vi "RunTest2.vi"(8 "error in (no error)":errorcluster, 11 "Prueba09 in":refnum<class "Prueba09.lvclass">) -> (0 "error out":errorcluster, 2 "resultado":string, 3 "Prueba09 out":refnum<class "Prueba09.lvclass">)   [LabVIEW 2019]
uses:
  <vilib>/Utility/miscctls.llb/LVRowAndColumnTypeDef.ctl
  Prueba/Prueba.lvclass
  Controles/Estados_P09.ctl
  Prueba09.lvclass
  Controles/MessageP09.ctl
  QMH/User Event - Stop/User Event - Stop.lvlib
  QMH/Message Queue/Message Queue.lvlib
  QMH/Message Queue/Enqueue Message (Single).vi
  ClusterGEN.ctl
  Prueba04/Control/Slide.ctl
  Prueba04/Prueba04.lvclass
  <vilib>/Utility/error.llb/Error Cluster From Error Code.vi
  <vilib>/ErrorRing/Error Ring.xnode
  <vilib>/Utility/error.llb/DialogType.ctl
  D:/REPO/GitHub/procal/Pruebas/Prueba/Prueba.lvclass
panel:
  out "elapsed time":dbl
  out "cuenta":i32
  out "tablaPeakRef[dB]":string[](array[string])
  out "Vref2":dbl
  out "Pict Ring 2":u16(ring)
  out "Pict Ring 3":u16(ring)
  out "cumple_no_cumple":bool
  out "Vref":dbl
  in  "Tab":enum32{"Page 1", "Page 2", "Page 3"}(tab)
  out "NivMaxCpeak":dbl=140.0
  out "NivelRMSensayo":dbl=95.0
  out "frecuencia1":dbl=140.0
  in  "guardar_Vref":bool
  in  "generar1":bool
  in  "AjusteAmp":T1 caption="Ajuste de amplitud [mV]" scale=0.0..100.0
  out "voltMon1":dbl format="%#.1f"
  out "frecMon1":dbl format="%#.1f"
  in  "seguir":bool
  out "NivMaxCpeak2":dbl=140.0
  out "NivelRMSensayo2":dbl=95.0
  out "frecuencia2":dbl=140.0
  in  "guardar_Vref2":bool
  in  "generar2":bool
  in  "AjusteAmp2":T1 caption="Ajuste de amplitud [mV]" scale=0.0..100.0
  out "voltMon2":dbl format="%#.1f"
  out "frecMon2":dbl format="%#.1f"
  in  "seguir2":bool
  out "Pict Ring 4":u16(ring)
  out "Pict Ring 1":u16(ring)
  out "led":bool
  in  "knobFrec":dbl(knob)=1.0 min=1.0 max=3.0 scale=1.0..3.0
  in  "genera3":bool caption="PruebaSup"
  out "voltMon500":dbl format="%#.1f"
  out "nivelRMS500":dbl format="%#.1f"
  in  "Tabla":string[][](table)
  in  "salir":bool
  out "cumple":bool
  out "no_cumple":bool
  out "voltMon8000":dbl format="%#.1f"
  out "nivelRM8000":dbl format="%#.1f"
  # "Selección de Señal de referencia 8000 Hz"
  # "Elección Señal de Referencia\nsegún marca y modelo de sonómetro"
  # "Nivel RMS para Ensayo"
  # "Nivel Máximo Cpeak"
  # "Frecuencia"
  # "Monitoreo"
  # "Frecuencia"
  # "Hz"
  # "Voltaje"
  # "mV"
  # "9. Nivel de sonido con ponderación Cpeak. IEC 61672-3: 2006 Cláusula 17"
  # "Selección de Señal de referencia 500 Hz"
  # "Elección Señal de Referencia\nsegún marca y modelo de sonómetro"
  # "Nivel RMS para Ensayo"
  # "Nivel Máximo Cpeak"
  # "Frecuencia"
  # "Monitoreo"
  # "Frecuencia"
  # "Hz"
  # "Voltaje"
  # "mV"
  # "9. Nivel de sonido con ponderación Cpeak. IEC 61672-3: 2006 Cláusula 17"
  # "Tabla Resultados"
  # "Genera peak"
  # "Cumple"
  # "No Cumple"
  # "500 Hz"
  # "Nivel RMS para Ensayo"
  # "dB"
  # "Voltaje"
  # "mV"
  # "9. Nivel de sonido con ponderación Cpeak. IEC 61672-3: 2006 Cláusula 17"
  # "8000 Hz"
  # "Nivel RMS para Ensayo"
  # "dB"
  # "Voltaje"
  # "mV"
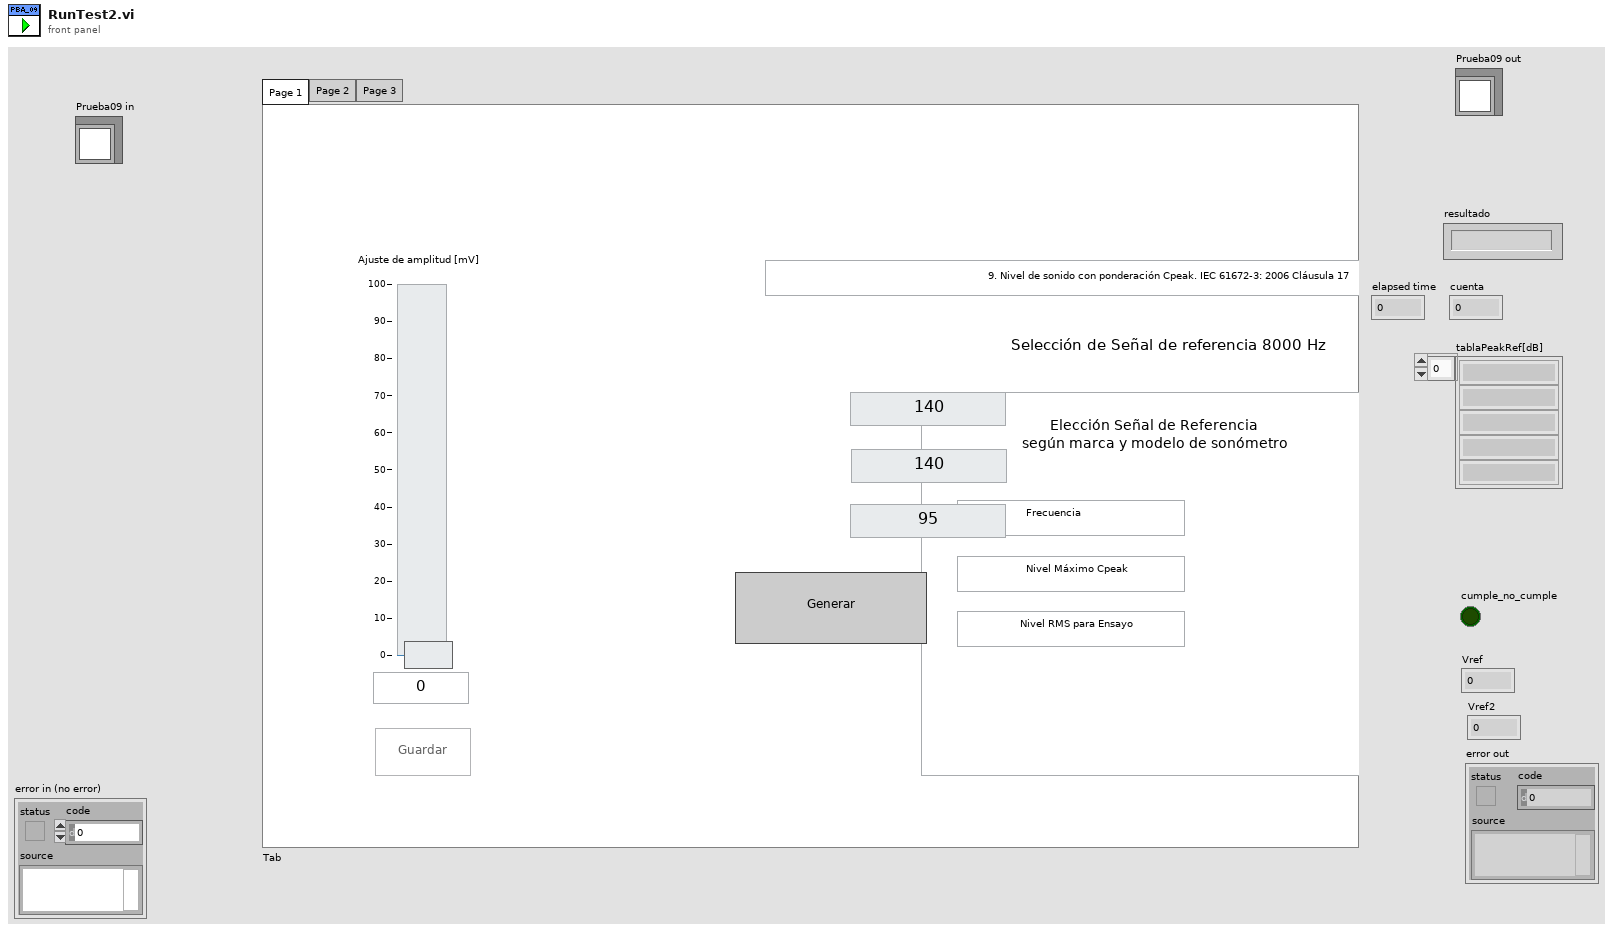
[diagram p1: front panel]
types:
  T1 = typedef "Prueba04.lvclass/Slide.ctl" = dbl
  T2 = typedef "LVRowAndColumnTypeDef.ctl" = cluster{"Row":i32, "Column":i32}
  T3 = typedef "Message Queue.lvlib/All Message Queues.ctl" = cluster{"MHL":refnum<queue>, "Inst_CNT90":refnum<queue>, "Inst_DS360":refnum<queue>, "Inst_Keithley2002":refnum<queue>, "Inst_DAQ":refnum<queue>, "BD":refnum<queue>, "Pistofono":refnum<queue>, "Nexus":refnum<queue>}
  T4 = enum8{"Enabled", "Disabled", "Disabled and Grayed Out"}
  T5 = enum32{"Page 1", "Page 2", "Page 3", "Page 4", "Page 5", "Page 6", "Page 7"}
  T6 = typedef "Prueba09.lvclass/ClusterGEN.ctl" = cluster{"frec":dbl, "amp":dbl, "tipo_ciclo":string}
  T7 = cluster{"ControlName":string, "ControlReference":refnum<vi>}[]
  T8 = typedef "Prueba09.lvclass/MessageP09.ctl" = cluster{"Estados":T9, "Data":variant}
  T9 = typedef "Prueba09.lvclass/Estados_P09.ctl" = enum16{"Error", "DetieneInstrumentos", "InicializarInstrumentos", "LeerArchivoConfiguracion", "inicio", "configurarTabla", "FrecAmp1", "FrecAmp2", "FrecAmp3", "iniciarGEN", "iniciaGEN_Peak", "detenerGEN", "guardaVref", "guardaVref2", "monitoreo", "peakRefer", "ingresaMediciones", "guardaMediciones", "cumplimiento", "listo_evaluar", "evaluar", "final", "salir"}
  T10 = typedef "DialogType.ctl" = u16
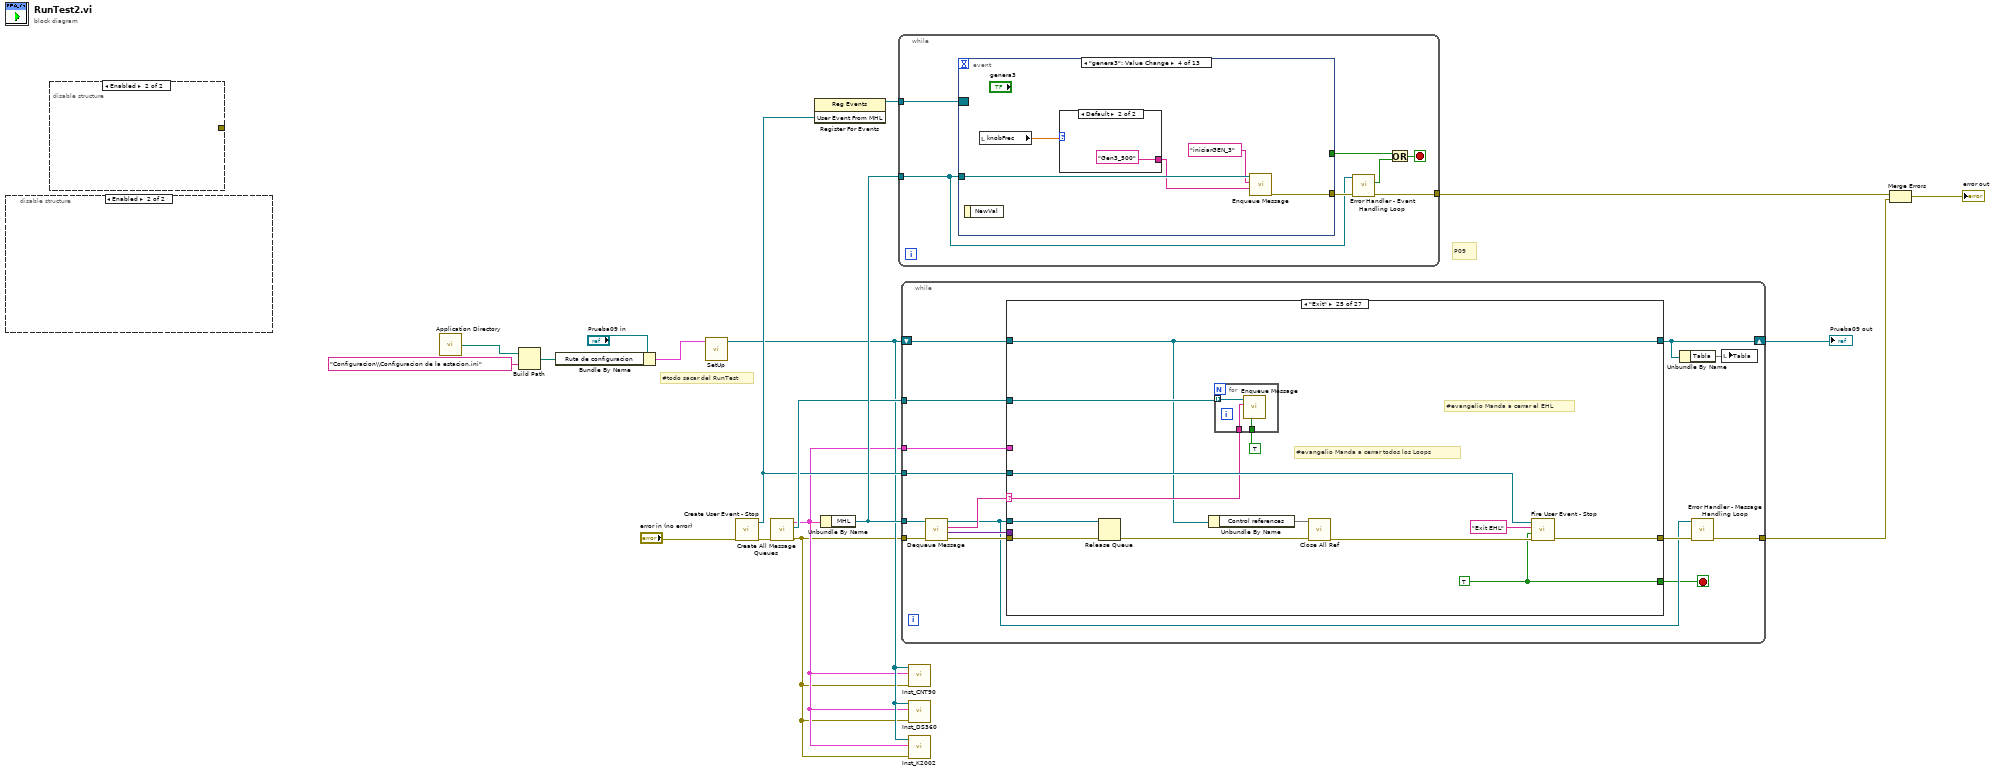
[diagram p0: block diagram]
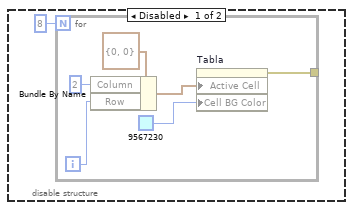
[diagram p2: hidden frame]
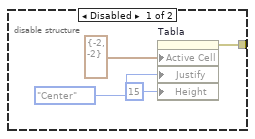
[diagram p3: hidden frame]
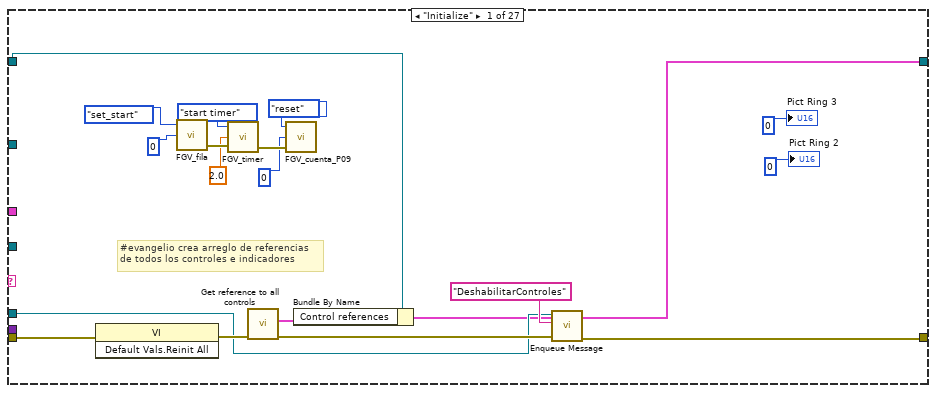
[diagram p4: hidden frame]
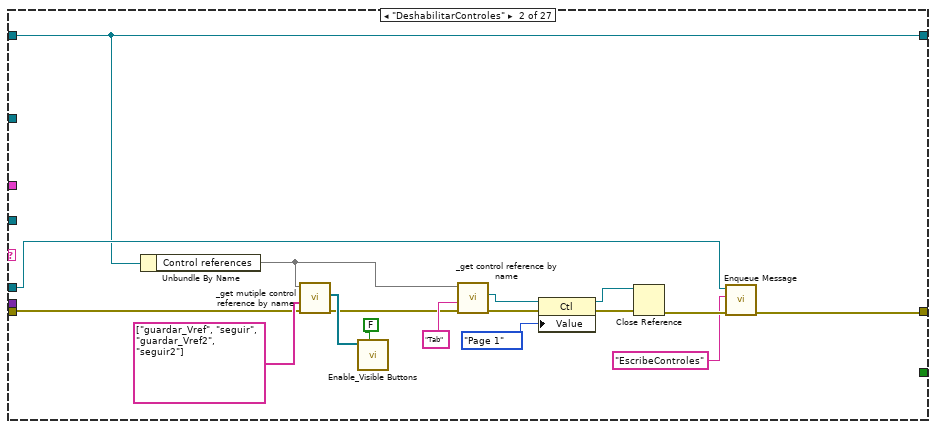
[diagram p5: hidden frame]
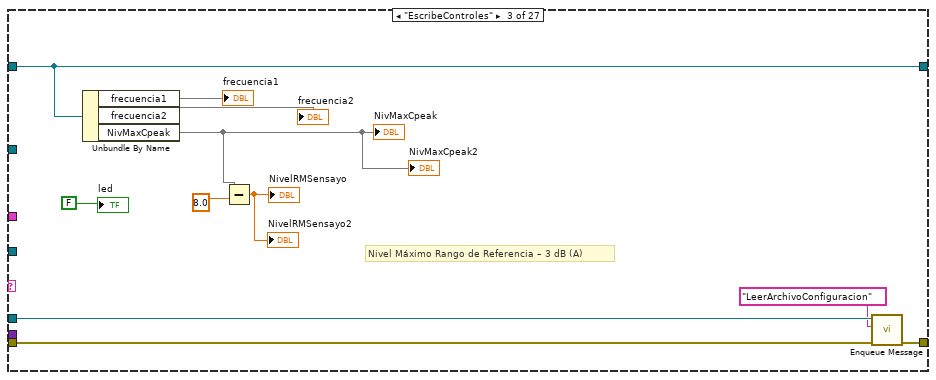
[diagram p6: hidden frame]
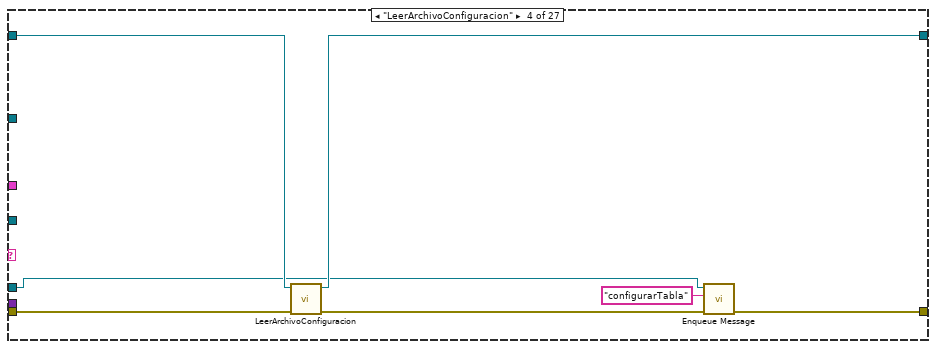
[diagram p7: hidden frame]
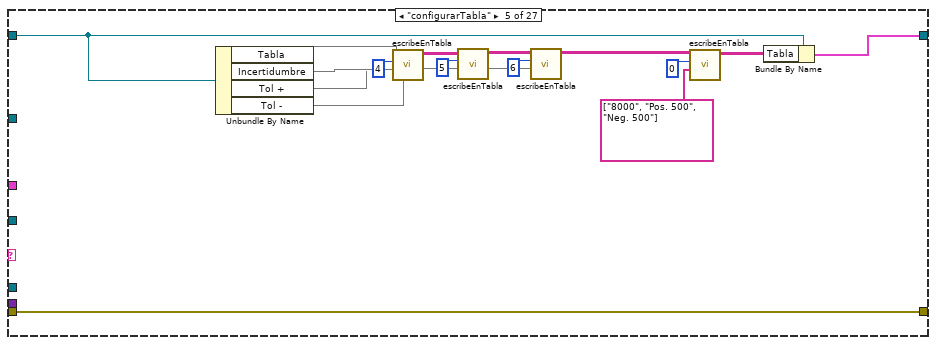
[diagram p8: hidden frame]
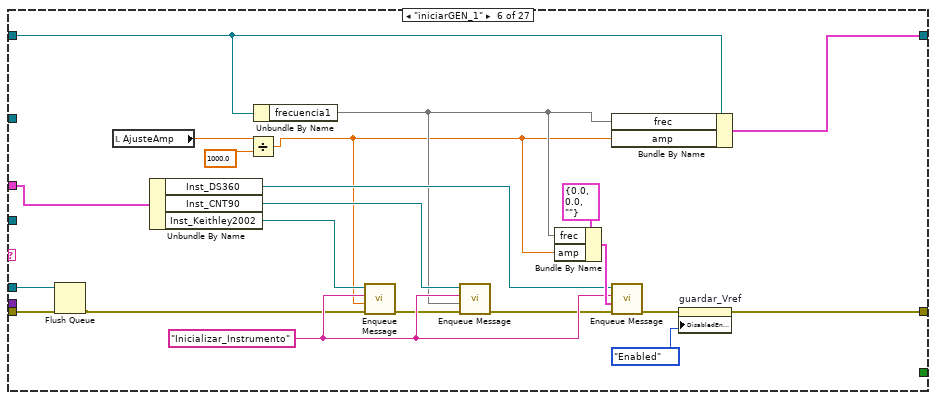
[diagram p9: hidden frame]
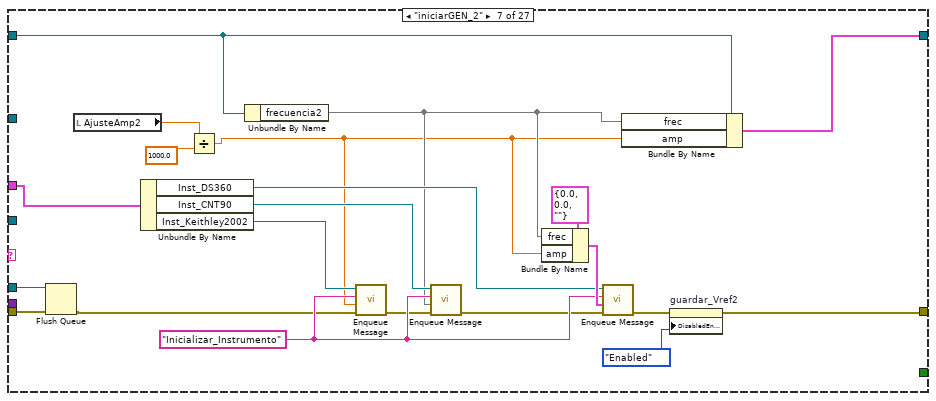
[diagram p10: hidden frame]
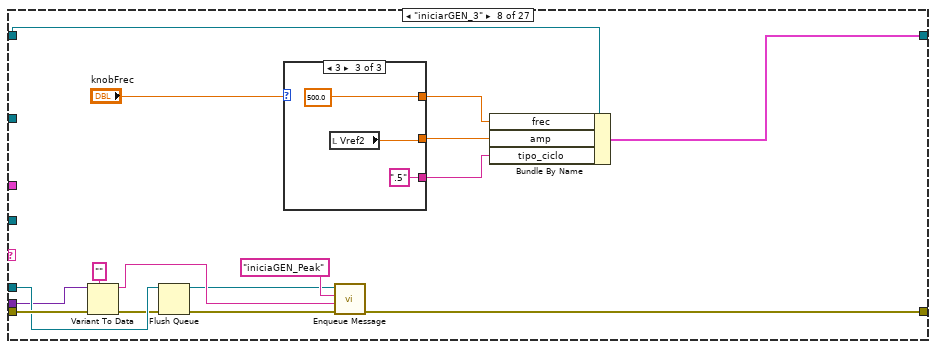
[diagram p11: hidden frame]
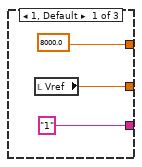
[diagram p12: hidden frame]
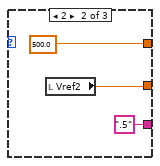
[diagram p13: hidden frame]
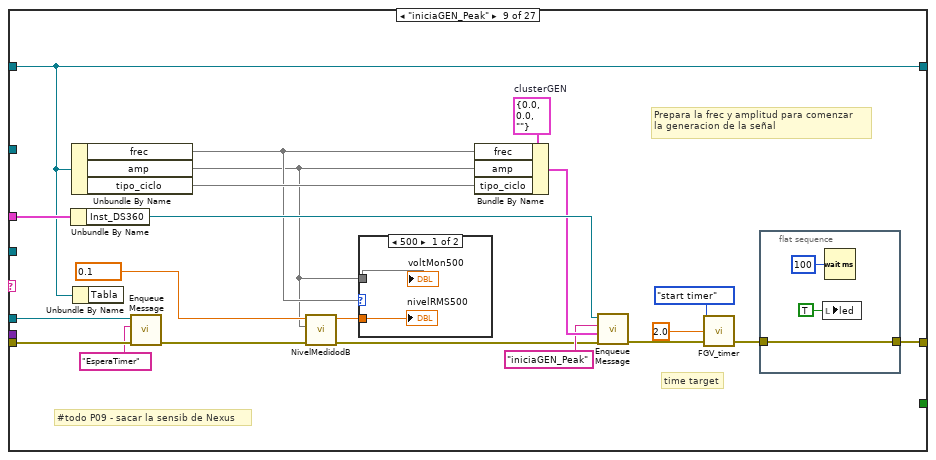
[diagram p14: hidden frame]
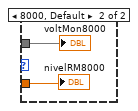
[diagram p15: hidden frame]
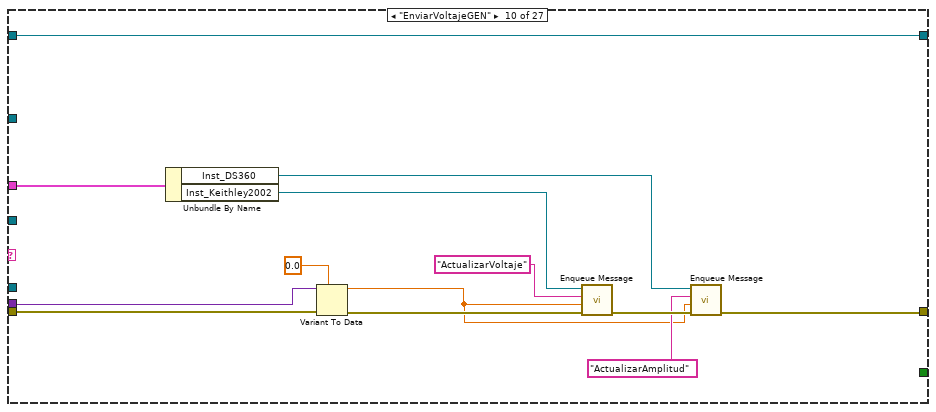
[diagram p16: hidden frame]
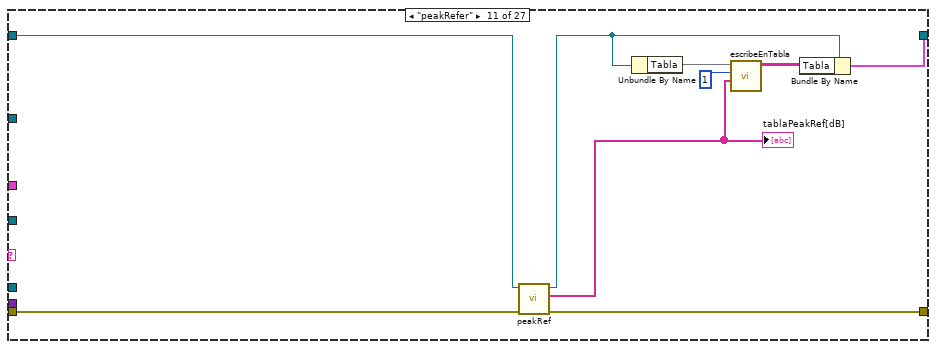
[diagram p17: hidden frame]
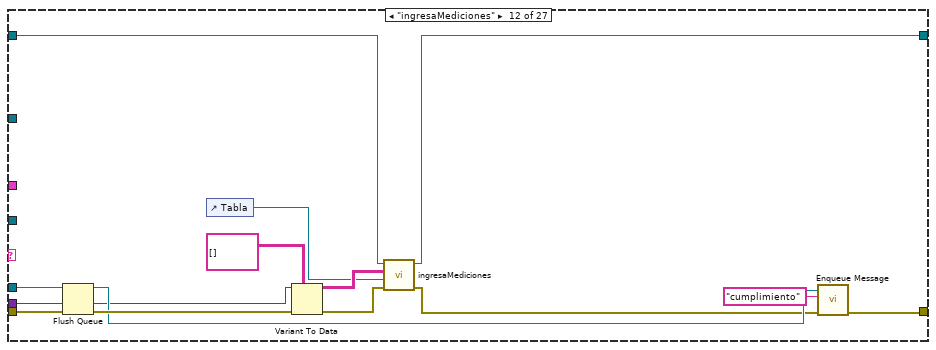
[diagram p18: hidden frame]
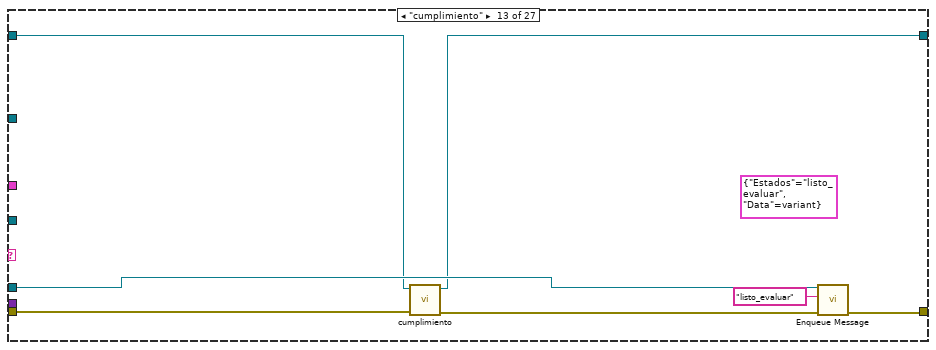
[diagram p19: hidden frame]
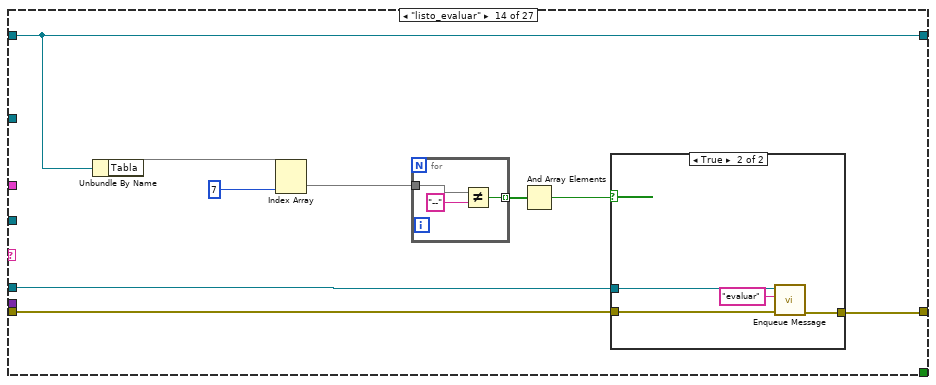
[diagram p20: hidden frame]
diagram:
  # "P09"
  # "#todo sacar del RunTest"
  n1 = disable-structure shown="Enabled" {
    frame Disabled {
      n2 = for {
        N: 8 -> [_]
        tunnel: [w21] -> _
        i -> [w20]
        n3 = Bundle By Name(cluster=T2 {"Row"=0, "Column"=0} ("Active Cell:Active Cell"), "Column"=2, "Row"=w20) -> (w23:T2)
        n4 = property on="Tabla" class="Tbl (strict)"("Active Cell"=w23, "Cell BG Color"=u32 9567230) -> (error out=w21:errorcluster)  [unwired: 2 in, 1 out]
      }
    }
    frame Enabled {
    }
  }
  n5 = disable-structure shown="Enabled" {
    disable-tunnel: [w28 _] -> _
    frame Disabled {
      n6 = property on="Tabla" class="Tbl (strict)"("Active Cell"=T2 {"Row"=-2, "Column"=-2} ("Active Cell:Active Cell"), "Justify"=enum16{"Left", "Center", "Right"}."Center" ("Active Cell:Cell Justification"), "Height"=u32 15 ("Active Cell:Cell Font:Size")) -> (error out=w28:errorcluster)  [unwired: 2 in, 1 out]
    }
    frame Enabled {
    }
  }
  n7 = call <vilib>:"Application Directory.vi"() -> ("Application Directory"=w14:path)
  n8 = Build Path(base path=w14, name or relative path="Configuracion\\Configuracion de la estacion.ini") -> (appended path=w11:path)
  n9 = Bundle By Name(cluster="Prueba09 in", "Ruta de configuracion"=w11) -> (w12:cluster{})
  n10 = call-dynamic "SetUp.vi"("Prueba08 in"=w12) -> ("Prueba08 out"=w3:refnum<class "Prueba09.lvclass">)  [unwired: 9 in, 1 out]
  n11 = call "Create User Event - Stop.vi"("error in (no error)"="error in (no error)") -> ("error out"=w9:errorcluster, "User Event From MHL"=w4:refnum<user-event>)  [unwired: 9 in]
  n12 = call "Create All Message Queues.vi"("error in (no error)"=w9) -> ("error out"=w1:errorcluster, "PL Queues Array"=w5:refnum<queue>[], "All Message Queues out"=w2:T3)  [unwired: 8 in]
  n13 = register-events(w4) -> (reference out=w6:refnum<event-registration>)  [unwired: 2 in, 1 out]
  n14 = Unbundle By Name(w2) -> ("MHL"=w7:refnum<queue>)
  n15 = while {
    tunnel: w7 -> [w31]
    tunnel: [w33] -> w18
    tunnel: w6 -> [w35]
    stop <- w36 stop-if-true
    n16 = event shown="[3] \"genera3\": Value Change" {
      selector: w35 -> [_ _ _ _ _ _ _ _ _ _ _ _ _]
      dyn-events: _ -> [_ _ _ _ _ _ _ _ _ _ _ _ _]
      timeout: _ -> [_ _ _ _ _ _ _ _ _ _ _ _ _]
      tunnel: w31 -> [w39 w44 w51 w55 _ w65 w70 w72 w81 w87 w91 _ w99]
      tunnel: [w38 w45 w50 w56 w60 w61 w71 w74 w78 w83 w90 _ _] -> w34
      tunnel: [_ _ _ _ _ _ _ _ _ _ _ w92 _] -> w30
      event "salir": Value Change {
        n17 = event-data() -> ()  [unwired: 1 in, 1 out]
        n18 = call-poly "Enqueue Message.vi"("Message"="Exit", "Message Queue"=w39) -> ("error out"=w38:errorcluster)  [unwired: 8 in, 1 out]
      }
      event "generar1": Value Change {
        n19 = event-data() -> ("NewVal"=w41:bool)  [unwired: 1 in]
        n20 = Select(t="iniciarGEN_1", s=w41, f="detenerGEN") -> (s? t:f=w40:string)
        n21 = call-poly "Enqueue Message.vi"("Message"=w40, "Message Queue"=w44) -> ("error out"=w45:errorcluster)  [unwired: 8 in, 1 out]
      }
      event "generar2": Value Change {
        n22 = event-data() -> ("NewVal"=w48:bool)  [unwired: 1 in]
        n23 = Select(t="iniciarGEN_2", s=w48, f="detenerGEN") -> (s? t:f=w46:string)
        n24 = call-poly "Enqueue Message.vi"("Message"=w46, "Message Queue"=w51) -> ("error out"=w50:errorcluster)  [unwired: 8 in, 1 out]
      }
      event "genera3": Value Change {
        n25 = event-data() -> ()  [unwired: 1 in, 1 out]
        n26 = local read "knobFrec"() -> (w54:dbl)
        n27 = case shown="Default" w54 {
          tunnel: ["Gen3_8000" "Gen3_500"] -> w52
          frame 1 {
          }
          frame Default {
          }
        }
        n28 = call-poly "Enqueue Message.vi"("Message Data"=w52, "Message"="iniciarGEN_3", "Message Queue"=w55) -> ("error out"=w56:errorcluster)  [unwired: 7 in, 1 out]
      }
      event "seguir": Value Change {
        n29 = event-data() -> ()  [unwired: 1 in, 1 out]
        n30 = property on="Tab" class="TabCtl (strict)"("Value"=enum32{"Page 1", "Page 2", "Page 3"}."Page 2" ("Tab")) -> (error out=w60:errorcluster)  [unwired: 2 in, 1 out]
      }
      event "seguir2": Value Change {
        n31 = event-data() -> ()  [unwired: 1 in, 1 out]
        n32 = call-poly "Enqueue Message.vi"("Message"="peakRefer", "Message Queue"=w65) -> ("error out"=w62:errorcluster)  [unwired: 8 in, 1 out]
        n33 = property on="Tab" class="TabCtl (strict)"(error in=w62, "Value"=enum32{"Page 1", "Page 2", "Page 3"}."Page 3" ("Tab")) -> (error out=w61:errorcluster)  [unwired: 1 in, 1 out]
      }
      event Value Change {
        n34 = event-data() -> ()  [unwired: 1 in, 1 out]
        n35 = Divide(x="AjusteAmp", y=T1 1000.0) -> (x/y=w66:T1)
        n36 = call-poly "Enqueue Message.vi"("Message Data"=w66, "Message"="EnviarVoltajeGEN", "Message Queue"=w70) -> ("error out"=w71:errorcluster)  [unwired: 7 in, 1 out]
      }
      event Value Change {
        n37 = event-data() -> ()  [unwired: 1 in, 1 out]
        n38 = Divide(x="AjusteAmp2", y=T1 1000.0) -> (x/y=w75:T1)
        n39 = call-poly "Enqueue Message.vi"("Message Data"=w75, "Message"="EnviarVoltajeGEN", "Message Queue"=w72) -> ("error out"=w74:errorcluster)  [unwired: 7 in, 1 out]
      }
      event "guardar_Vref": Value Change {
        n40 = event-data() -> ()  [unwired: 1 in, 1 out]
        n41 = call-poly "Enqueue Message.vi"("Message"="guardaVref", "Message Queue"=w81) -> ("error out"=w79:errorcluster)  [unwired: 8 in, 1 out]
        n42 = property on="seguir" class="Bool"(error in=w79, "DisabledEnum"=T4."Enabled" ("Disabled")) -> (error out=w78:errorcluster)  [unwired: 1 in, 1 out]
      }
      event "guardar_Vref2": Value Change {
        n43 = event-data() -> ()  [unwired: 1 in, 1 out]
        n44 = call-poly "Enqueue Message.vi"("Message"="guardaVref2", "Message Queue"=w87) -> ("error out"=w84:errorcluster)  [unwired: 8 in, 1 out]
        n45 = property on="seguir2" class="Bool"(error in=w84, "DisabledEnum"=T4."Enabled" ("Disabled")) -> (error out=w83:errorcluster)  [unwired: 1 in, 1 out]
      }
      event "Tabla": Value Change {
        n46 = event-data() -> ("NewVal"=w89:string[][])  [unwired: 1 in]
        n47 = call-poly "Enqueue Message.vi"("Message Data"=w89, "Message"="ingresaMediciones", "Message Queue"=w91) -> ("error out"=w90:errorcluster)  [unwired: 7 in, 1 out]
      }
      event User Event {
        n48 = event-data() -> ("User Event"=w94:string, "Event Data"=w93:variant)  [unwired: 1 in]
        n49 = case shown="\"Exit EHL\"" w94 {
          tunnel: w93 -> [_ w96]
          tunnel: [_ w95] -> w92
          frame Default {
          }
          frame "Exit EHL" {
            # "#evangelio Termina\nla ejecucion del EHL"
            n50 = Variant To Data(type=TRUE, Variant=w96) -> (data=w95:bool)  [unwired: 1 in, 1 out]
          }
        }
      }
      event Panel Close? {
        w98 = TRUE
        n51 = event-data() -> ()  [unwired: 1 in, 1 out]
        n52 = call-poly "Enqueue Message.vi"("Priority Message? (F)"=w98, "Message"="Confirmar Salida", "Message Queue"=w99) -> ()  [unwired: 7 in, 2 out]
        n53 = event-data("Discard?"=w98) -> ()  [unwired: 1 in, 1 out]
      }
    }
    n54 = call "Error Handler - Event Handling Loop.vi"("error in (no error)"=w34, "Message Queue"=w31) -> ("dup error in"=w33:errorcluster, "Error?"=w32:bool)  [unwired: 7 in, 1 out]
    n55 = Or(x=w30, y=w32) -> (x .or. y?=w36:bool)
  }
  n56 = while {
    tunnel: w7 -> [w109]
    tunnel: w1 -> [w108]
    tunnel: [w103] -> w10
    shift-right: [w114] -> w16
    shift-left: w3 -> [w115]
    tunnel: w2 -> [w112]
    tunnel: w5 -> [w111]
    tunnel: w4 -> [w110]
    stop <- w101 stop-if-true
    n57 = call "Dequeue Message.vi"("error in (no error)"=w108, "Message Queue"=w109) -> ("error out"=w107:errorcluster, "Message Data"=w105:variant, "Message"=w106:string, "dup Message Queue"=w102:refnum<queue>)  [unwired: 6 in]
    n58 = case shown="\"Exit\"" w106 {
      selector: w106 -> [_ _ _ _ _ _ _ _ _ _ _ _ _ _ _ _ _ _ _ _ _ _ _ _ w470 _ w497]
      tunnel: w105 -> [_ _ _ _ _ _ _ w233 _ w283 _ w310 _ _ _ _ _ w407 w416 _ _ _ w455 _ _ _ _]
      tunnel: w107 -> [w129 w138 w162 w169 w179 w195 w215 w243 w273 w284 w302 w316 w323 w332 w348 w359 w363 w408 w417 w422 w441 w448 w458 w466 w474 w485 _]
      tunnel: [w128 w135 w161 w165 w179 w193 w211 w242 w268 w281 w301 w315 w321 w331 w346 w359 w374 w402 w412 w418 w441 w448 w456 w466 w468 w483 w496] -> w104
      tunnel: w102 -> [w130 w137 w160 w164 _ w194 w214 w240 w260 _ _ w313 w320 w330 w347 _ w362 _ _ w421 _ _ w457 _ w473 w484 _]
      tunnel: w115 -> [w117 w136 w158 w167 w176 w205 w226 w238 w255 w293 w300 w308 w319 w325 w343 w354 w361 w406 w415 w419 w442 w449 w464 w465 w469 w490 w498]
      tunnel: [w116 w136 w158 w168 w175 w206 w227 w239 w255 w293 w295 w307 w318 w325 w343 w354 w361 w405 w414 w419 w442 w449 w464 w465 w469 w490 w498] -> w114
      tunnel: w112 -> [_ _ _ _ _ w192 w213 _ w267 w282 _ _ _ _ _ _ _ _ _ w420 _ _ _ _ _ _ _]
      tunnel: w111 -> [_ _ _ _ _ _ _ _ _ _ _ _ _ _ _ _ _ _ _ _ _ _ _ _ w472 _ _]
      tunnel: w110 -> [_ _ _ _ _ _ _ _ _ _ _ _ _ _ _ _ _ _ _ _ _ _ _ _ w471 _ _]
      tunnel: [_ _ _ _ _ _ _ _ _ _ _ _ _ _ _ _ _ _ _ _ _ _ _ _ w467 _ _] -> w101
      frame "Initialize" {
        # "#evangelio crea arreglo de referencias\nde todos los controles e indicadores"
        n59 = invoke class="VI" method="Default Vals.Reinit All"(error in=w129) -> (error out=w133:errorcluster)  [unwired: 2 in, 2 out]
        n60 = call "FGV_fila.vi"("fila_inicial"=0, "action"=enum16{"increment", "set_start", "get"}."set_start") -> ("error out"=w127:errorcluster)  [unwired: 2 in, 1 out]
        n61 = call "FGV_timer.vi"("error in (no error)"=w127, "time target"=2.0, "action"=enum16{"get time", "start timer"}."start timer") -> ("error out"=w126:errorcluster)  [unwired: 2 out]
        n62 = call "Get reference to all controls.vi"("error in (no error)"=w133) -> ("error out"=w131:errorcluster, "Control references"=w132:T7)  [unwired: 5 in]
        n63 = call "FGV_cuenta_P09.vi"("error in (no error)"=w126, "cuenta in"=0, "action"=enum16{"increment", "reset", "get"}."reset") -> ()  [unwired: 1 in, 2 out]
        n64 = Bundle By Name(cluster=w117, "Control references"=w132) -> (w116:cluster{})
        n65 = call-poly "Enqueue Message.vi"("error in (no error)"=w131, "Message"="DeshabilitarControles", "Message Queue"=w130) -> ("error out"=w128:errorcluster)  [unwired: 7 in, 1 out]
        "Pict Ring 2" <- u16 0 ("Pict Ring 2")
        "Pict Ring 3" <- u16 0 ("Pict Ring 3")
      }
      frame "DeshabilitarControles" {
        n66 = Unbundle By Name(w136) -> ("Control references"=w147)
        n67 = call "_get mutiple control reference by name.vi"("error in (no error)"=w138, "Control names"=string[] ["guardar_Vref", "seguir", "guardar_Vref2", "seguir2"], "Control references"=w147) -> ("error out"=w144:errorcluster, "References"=w145:refnum<vi>[])  [unwired: 3 in]
        n68 = call "Enable_Visible Buttons.vi"("Enable? (T)"=FALSE, "Controls Ref Array"=w145) -> ()  [unwired: 10 in]
        n69 = call "_get control reference by name.vi"("error in (no error)"=w144, "Control name"="Tab" ("Message"), "Control references"=w147) -> ("error out"=w151:errorcluster, "Ctl Refnum"=w149:refnum<vi>)  [unwired: 3 in]
        n70 = property class="Ctl"(reference=w149, error in=w151, "Value"=T5."Page 1" ("Tab_Prueba04")) -> (reference out=w140:refnum<vi>, error out=w142:errorcluster)
        n71 = Close Reference(reference=w140, error in (no error)=w142) -> (error out=w141:errorcluster)
        n72 = call-poly "Enqueue Message.vi"("error in (no error)"=w141, "Message"="EscribeControles", "Message Queue"=w137) -> ("error out"=w135:errorcluster)  [unwired: 7 in, 1 out]
      }
      frame "EscribeControles" {
        # "Nivel Máximo Rango de Referencia – 3 dB (A)"
        n73 = Unbundle By Name(w158) -> ("frecuencia1"=→"frecuencia1", "frecuencia2"=→"frecuencia2", "NivMaxCpeak"=w155)
        "NivMaxCpeak" <- w155
        "NivMaxCpeak2" <- w155
        n74 = Subtract(x=w155, y=8.0) -> (x-y=→"NivelRMSensayo" →"NivelRMSensayo2":dbl)
        n75 = call-poly "Enqueue Message.vi"("error in (no error)"=w162, "Message"="LeerArchivoConfiguracion", "Message Queue"=w160) -> ("error out"=w161:errorcluster)  [unwired: 7 in, 1 out]
        "led" <- FALSE ("led")
      }
      frame "LeerArchivoConfiguracion" {
        n76 = call "LeerArchivoConfiguracion.vi"("error in"=w169, "Prueba31 in"=w167) -> ("error out"=w166:errorcluster, "Prueba31 out"=w168:refnum<class "Prueba09.lvclass">)  [unwired: 8 in]
        n77 = call-poly "Enqueue Message.vi"("error in (no error)"=w166, "Message"="configurarTabla", "Message Queue"=w164) -> ("error out"=w165:errorcluster)  [unwired: 7 in, 1 out]
      }
      frame "configurarTabla" {
        n78 = Unbundle By Name(w176) -> ("Tabla"=w174, "Incertidumbre"=w173, "Tol +"=w172, "Tol -"=w171)
        n79 = call "escribeEnTabla.vi"("parametros"=w173, "col"=4, "tabla in"=w174) -> ("tabla out"=w185:string[][])  [unwired: 8 in]
        n80 = call "escribeEnTabla.vi"("parametros"=w172, "col"=5, "tabla in"=w185) -> ("tabla out"=w184:string[][])  [unwired: 8 in]
        n81 = call "escribeEnTabla.vi"("parametros"=w171, "col"=6, "tabla in"=w184) -> ("tabla out"=w180:string[][])  [unwired: 8 in]
        n82 = call "escribeEnTabla.vi"("parametros"=string[] ["8000", "Pos. 500", "Neg. 500"], "col"=0, "tabla in"=w180) -> ("tabla out"=w178:string[][])  [unwired: 8 in]
        n83 = Bundle By Name(cluster=w176, "Tabla"=w178) -> (w175:cluster{})
      }
      frame "iniciarGEN_1" {
        w202 = "Inicializar_Instrumento" ("Message")
        n84 = Flush Queue(queue=w194, error in (no error)=w195) -> (error out=w197:errorcluster)  [unwired: 2 out]
        n85 = local read "AjusteAmp"() -> (w188:T1)
        n86 = Unbundle By Name(w192) -> ("Inst_DS360"=w190:refnum<queue>, "Inst_CNT90"=w196:refnum<queue>, "Inst_Keithley2002"=w204:refnum<queue>)
        n87 = Divide(x=w188, y=T1 1000.0) -> (x/y=w186:T1)
        n88 = Unbundle By Name(w205) -> ("frecuencia1"=w189)
        n89 = call-poly "Enqueue Message.vi"("error in (no error)"=w197, "Message Data"=w186, "Message"=w202, "Message Queue"=w204) -> ("error out"=w201:errorcluster)  [unwired: 6 in, 1 out]
        n90 = call-poly "Enqueue Message.vi"("error in (no error)"=w201, "Message Data"=w189, "Message"=w202, "Message Queue"=w196) -> ("error out"=w200:errorcluster)  [unwired: 6 in, 1 out]
        n91 = Bundle By Name(cluster=T6 {"frec"=0.0, "amp"=0.0, "tipo_ciclo"=""} ("clusterGEN"), "frec"=w189, "amp"=w186) -> (w203:T6)
        n92 = Bundle By Name(cluster=w205, "frec"=w189, "amp"=w186) -> (w206:cluster{})
        n93 = call-poly "Enqueue Message.vi"("error in (no error)"=w200, "Message Data"=w203, "Message"=w202, "Message Queue"=w190) -> ("error out"=w198:errorcluster)  [unwired: 6 in, 1 out]
        n94 = property on="guardar_Vref" class="Bool"(error in=w198, "DisabledEnum"=T4."Enabled" ("Disabled")) -> (error out=w193:errorcluster)  [unwired: 1 in, 1 out]
      }
      frame "iniciarGEN_2" {
        w223 = "Inicializar_Instrumento" ("Message")
        n95 = Flush Queue(queue=w214, error in (no error)=w215) -> (error out=w217:errorcluster)  [unwired: 2 out]
        n96 = local read "AjusteAmp2"() -> (w209:T1)
        n97 = Unbundle By Name(w213) -> ("Inst_DS360"=w218:refnum<queue>, "Inst_CNT90"=w216:refnum<queue>, "Inst_Keithley2002"=w225:refnum<queue>)
        n98 = Divide(x=w209, y=T1 1000.0) -> (x/y=w207:T1)
        n99 = Unbundle By Name(w226) -> ("frecuencia2"=w210)
        n100 = call-poly "Enqueue Message.vi"("error in (no error)"=w217, "Message Data"=w207, "Message"=w223, "Message Queue"=w225) -> ("error out"=w222:errorcluster)  [unwired: 6 in, 1 out]
        n101 = call-poly "Enqueue Message.vi"("error in (no error)"=w222, "Message Data"=w210, "Message"=w223, "Message Queue"=w216) -> ("error out"=w221:errorcluster)  [unwired: 6 in, 1 out]
        n102 = Bundle By Name(cluster=T6 {"frec"=0.0, "amp"=0.0, "tipo_ciclo"=""} ("clusterGEN"), "frec"=w210, "amp"=w207) -> (w224:T6)
        n103 = call-poly "Enqueue Message.vi"("error in (no error)"=w221, "Message Data"=w224, "Message"=w223, "Message Queue"=w218) -> ("error out"=w219:errorcluster)  [unwired: 6 in, 1 out]
        n104 = Bundle By Name(cluster=w226, "frec"=w210, "amp"=w207) -> (w227:cluster{})
        n105 = property on="guardar_Vref2" class="Bool"(error in=w219, "DisabledEnum"=T4."Enabled" ("Disabled")) -> (error out=w211:errorcluster)  [unwired: 1 in, 1 out]
      }
      frame "iniciarGEN_3" {
        n106 = Variant To Data(error in=w243, type="", Variant=w233) -> (data=w229:string, error out=w234:errorcluster)
        n107 = Flush Queue(queue=w240, error in (no error)=w234) -> (queue out=w228:refnum<queue>, error out=w241:errorcluster)  [unwired: 1 out]
        n108 = case shown="3" "knobFrec" {
          tunnel: [8000.0 500.0 500.0] -> w236
          tunnel: [w245 w248 w251] -> w235
          tunnel: ["1" ("tipo_ciclo") ".5" ("tipo_ciclo") ".5" ("tipo_ciclo")] -> w231
          frame 1, Default {
            n109 = local read "Vref"() -> (w245:dbl)
          }
          frame 2 {
            n110 = local read "Vref2"() -> (w248:dbl)
          }
          frame 3 {
            n111 = local read "Vref2"() -> (w251:dbl)
          }
        }
        n112 = call-poly "Enqueue Message.vi"("error in (no error)"=w241, "Message Data"=w229, "Message"="iniciaGEN_Peak" ("tipo_ciclo"), "Message Queue"=w228) -> ("error out"=w242:errorcluster)  [unwired: 6 in, 1 out]
        n113 = Bundle By Name(cluster=w238, "frec"=w236, "amp"=w235, "tipo_ciclo"=w231) -> (w239:cluster{})
      }
      frame "iniciaGEN_Peak" {
        w254 = 0.1 items=["10m"=0.01, "31,6m"=0.0316, "100m"=0.1, "316m"=0.316, "1"=1.0] ("Sensibilidad")
        w265 = T6 {"frec"=0.0, "amp"=0.0, "tipo_ciclo"=""}  # clusterGEN
        # "#todo P09 - sacar la sensib de Nexus"
        # "time target"
        # "Prepara la frec y amplitud para comenzar\nla generacion de la señal"
        n114 = Unbundle By Name(w267) -> ("Inst_DS360"=w266:refnum<queue>)
        n115 = Unbundle By Name(w255) -> ("frec"=w256, "amp"=w253, "tipo_ciclo"=w264)
        n116 = Unbundle By Name(w255) -> ()  [unwired: 1 out]
        n117 = call-poly "Enqueue Message.vi"("error in (no error)"=w273, "Message"="EsperaTimer", "Message Queue"=w260) -> ("error out"=w261:errorcluster)  [unwired: 7 in, 1 out]
        n118 = call "NivelMedidodB.vi"("error in (no error)"=w261, "voltaje_medido"=w253, "Sensibilidad"=w254) -> ("error out"=w258:errorcluster, "Nivel Medido [dB]"=w257:dbl)  [unwired: 7 in]
        n119 = case shown="500" w256 {
          tunnel: w257 -> [w275 w277]
          tunnel: w253 -> [w274 w276]
          frame 500 {
            "nivelRMS500" <- w275
            "voltMon500" <- w274
          }
          frame 8000, Default {
            "voltMon8000" <- w276
            "nivelRM8000" <- w277
          }
        }
        n120 = Bundle By Name(cluster=w265, "frec"=w256, "amp"=w253, "tipo_ciclo"=w264) -> (w263:T6)
        n121 = call-poly "Enqueue Message.vi"("error in (no error)"=w258, "Message Data"=w263, "Message"="iniciaGEN_Peak", "Message Queue"=w266) -> ("error out"=w272:errorcluster)  [unwired: 6 in, 1 out]
        n122 = call "FGV_timer.vi"("error in (no error)"=w272, "time target"=2.0, "action"=enum16{"get time", "start timer"}."start timer") -> ("error out"=w269:errorcluster)  [unwired: 2 out]
        n123 = flat-sequence {
          tunnel: w269 -> [w280]
          tunnel: [w280] -> w268
          frame #0 {
            n124 = local write "led"(TRUE ("led")) -> ()
            n125 = Wait (ms)(milliseconds to wait=u32 100) -> ()  [unwired: 1 out]
          }
        }
      }
      frame "EnviarVoltajeGEN" {
        n126 = Unbundle By Name(w282) -> ("Inst_DS360"=w287:refnum<queue>, "Inst_Keithley2002"=w292:refnum<queue>)
        n127 = Variant To Data(error in=w284, type=0.0, Variant=w283) -> (data=w285:dbl, error out=w290:errorcluster)
        n128 = call-poly "Enqueue Message.vi"("error in (no error)"=w290, "Message Data"=w285, "Message"="ActualizarVoltaje", "Message Queue"=w292) -> ("error out"=w288:errorcluster)  [unwired: 6 in, 1 out]
        n129 = call-poly "Enqueue Message.vi"("error in (no error)"=w288, "Message Data"=w285, "Message"="ActualizarAmplitud", "Message Queue"=w287) -> ("error out"=w281:errorcluster)  [unwired: 6 in, 1 out]
      }
      frame "peakRefer" {
        n130 = call "peakRef.vi"("error in (no error)"=w302, "Prueba09 in"=w300) -> ("error out"=w301:errorcluster, "tablaPeakRef[dB]"=w296:string[], "Prueba09 out"=w299:refnum<class "Prueba09.lvclass">)  [unwired: 7 in]
        "tablaPeakRef[dB]" <- w296
        n131 = Unbundle By Name(w299) -> ("Tabla"=w298)
        n132 = call "escribeEnTabla.vi"("parametros"=w296, "col"=1, "tabla in"=w298) -> ("tabla out"=w294:string[][])  [unwired: 8 in]
        n133 = Bundle By Name(cluster=w299, "Tabla"=w294) -> (w295:cluster{})
      }
      frame "ingresaMediciones" {
        n134 = Flush Queue(queue=w313, error in (no error)=w316) -> (queue out=w312:refnum<queue>, error out=w314:errorcluster)  [unwired: 1 out]
        n135 = control-ref of="Tabla"() -> (w305:refnum<vi>)
        n136 = Variant To Data(error in=w314, type=string[][] [] ("NewVal"), Variant=w310) -> (data=w306:string[][], error out=w309:errorcluster)
        n137 = call "ingresaMediciones.vi"("error in (no error)"=w309, 9:w305, "Selection Start"=w306, "Prueba09 in"=w308) -> ("error out"=w304:errorcluster, "Prueba09 out"=w307:refnum<class "Prueba09.lvclass">)  [unwired: 6 in]
        n138 = call-poly "Enqueue Message.vi"("error in (no error)"=w304, "Message"="cumplimiento", "Message Queue"=w312) -> ("error out"=w315:errorcluster)  [unwired: 7 in, 1 out]
      }
      frame "cumplimiento" {
        (unwired) T8 {"Estados"=enum."listo_evaluar", "Data"=variant} ("element")
        n139 = call "cumplimiento.vi"("error in (no error)"=w323, "Prueba09 in"=w319) -> ("error out"=w322:errorcluster, "Prueba09 out"=w318:refnum<class "Prueba09.lvclass">)  [unwired: 8 in]
        n140 = call-poly "Enqueue Message.vi"("error in (no error)"=w322, "Message"="listo_evaluar", "Message Queue"=w320) -> ("error out"=w321:errorcluster)  [unwired: 7 in, 1 out]
      }
      frame "listo_evaluar" {
        n141 = Unbundle By Name(w325) -> ("Tabla"=w324)
        n142 = Index Array(array=w324, index (col)=7 ("disabled index (col)")) -> (element=w327)  [unwired: 1 in]
        n143 = for {
          tunnel: [w340] -> w328 mode=indexing
          tunnel: w327 -> [w338]
          n144 = Not Equal?(x=w338, y="--") -> (x != y?=w340:bool)
        }
        n145 = And Array Elements(Boolean array=w328) -> (logical AND=w326:bool)
        n146 = case shown="True" w326 {
          tunnel: w332 -> [w333 w337]
          tunnel: [w333 w336] -> w331
          tunnel: w330 -> [_ w335]
          frame False {
          }
          frame True {
            n147 = call-poly "Enqueue Message.vi"("error in (no error)"=w337, "Message"="evaluar", "Message Queue"=w335) -> ("error out"=w336:errorcluster)  [unwired: 7 in, 1 out]
          }
        }
      }
      frame "evaluar" {
        # "si todos cumplen\nentonces el ensayo\ncumple"
        n148 = Unbundle By Name(w343) -> ("Tabla"=w342)
        n149 = call-poly "Enqueue Message.vi"("error in (no error)"=w348, "Message"="final", "Message Queue"=w347) -> ("error out"=w346:errorcluster)  [unwired: 7 in, 1 out]
        n150 = Index Array(array=w342, index (col)=7 ("disabled index (col)")) -> (element=w344)  [unwired: 1 in]
        n151 = for {
          tunnel: [w353] -> w350 mode=indexing
          tunnel: w344 -> [w351]
          n152 = Equal?(x=w351, y="Cumple") -> (x = y?=w353:bool)
        }
        n153 = And Array Elements(Boolean array=w350) -> (logical AND=→"cumple_no_cumple":bool)
      }
      frame "final" {
        n154 = local read "cumple_no_cumple"() -> (w355:bool)
        "cumple" <- w355
        n155 = Not(x=w355) -> (.not. x?=→"no_cumple":bool)
        n156 = Select(t="Cumple", s=w355, f="No Cumple") -> (s? t:f=→"resultado":string)
      }
      frame "EsperaTimer" {
        n157 = call "FGV_timer.vi"("error in (no error)"=w363, "time target"=2.0, "action"=enum16{"get time", "start timer"}."get time") -> ("error out"=w371:errorcluster, "time elapsed?"=w372:bool, "elapsed time"=→"elapsed time":dbl)
        n158 = call "FGV_cuenta_P09.vi"("error in (no error)"=w371, "action"=enum16{"increment", "reset", "get"}."get") -> ("error out"=w364:errorcluster, "cuenta out"=w370:i32)  [unwired: 2 in]
        "cuenta" <- w370
        n159 = Greater Or Equal?(x=w370, y=9) -> (x >= y?=w368:bool)
        n160 = case shown="True" w372 {
          tunnel: [w380 w381] -> w374
          tunnel: w364 -> [w379 w387]
          tunnel: w368 -> [_ w386]
          tunnel: w362 -> [w378 w383]
          frame False {
            # "Aun no llegamos a los 2 segundos"
            n161 = call-poly "Enqueue Message.vi"("error in (no error)"=w379, "Message"="EsperaTimer", "Message Queue"=w378) -> ("error out"=w380:errorcluster)  [unwired: 7 in, 1 out]
            n162 = local write "led"(FALSE ("led")) -> ()
            n163 = Wait (ms)(milliseconds to wait=u32 250) -> ()  [unwired: 1 out]
          }
          frame True {
            # "Pasamos los 2 segundos"
            n164 = case shown="False" w386 {
              tunnel: [w389 w396] -> w382
              tunnel: w387 -> [w395 w401]
              tunnel: w383 -> [w392 w399]
              frame True {
                # "Pasamos los 10 pulsos"
                n165 = local write "genera3"(FALSE ("genera3")) -> ()
                n166 = call-poly "Enqueue Message.vi"("error in (no error)"=w395, "Message"="detenerGEN", "Message Queue"=w392) -> ("error out"=w390:errorcluster)  [unwired: 7 in, 1 out]
                n167 = call "FGV_cuenta_P09.vi"("error in (no error)"=w390, "cuenta in"=0, "action"=enum16{"increment", "reset", "get"}."reset") -> ("error out"=w389:errorcluster)  [unwired: 1 in, 1 out]
              }
              frame False {
                # "aun no llegamos a los 10 pulsos"
                n168 = call-poly "Enqueue Message.vi"("error in (no error)"=w401, "Message"="iniciaGEN_Peak", "Message Queue"=w399) -> ("error out"=w397:errorcluster)  [unwired: 7 in, 1 out]
                n169 = call "FGV_cuenta_P09.vi"("error in (no error)"=w397, "action"=enum16{"increment", "reset", "get"}."increment") -> ("error out"=w396:errorcluster)  [unwired: 2 in, 1 out]
              }
            }
            n170 = call "FGV_timer.vi"("error in (no error)"=w382, "time target"=2.0, "action"=enum16{"get time", "start timer"}."start timer") -> ("error out"=w381:errorcluster)  [unwired: 2 out]
          }
        }
      }
      frame "DatoRecibidoCNT90" {
        n171 = Variant To Data(error in=w408, type=0.0, Variant=w407) -> (data=w403:dbl, error out=w402:errorcluster)
        "frecMon2" <- w403
        "frecMon1" <- w403
        n172 = Bundle By Name(cluster=w406, "frecMedida"=w403) -> (w405:cluster{})
      }
      frame "DatoRecibidoK2002" {
        n173 = Variant To Data(error in=w417, type=0.0, Variant=w416) -> (data=w410:dbl, error out=w412:errorcluster)
        n174 = Multiply(x=w410, y=1000.0) -> (x*y=w409:dbl)
        "voltMon2" <- w409
        "voltMon1" <- w409
        n175 = Bundle By Name(cluster=w415, "voltMedido"=w409) -> (w414:cluster{})
      }
      frame "detenerGEN" {
        w435 = TRUE ("Priority Message? (F)")
        w436 = "Detener_Instrumento"
        w440 = 0.0 ("voltaje1")
        n176 = Unbundle By Name(w420) -> ("Inst_DS360"=w437:refnum<queue>, "Inst_CNT90"=w438:refnum<queue>, "Inst_Keithley2002"=w439:refnum<queue>)
        n177 = Flush Queue(queue=w421, error in (no error)=w422) -> (error out=w424:errorcluster)  [unwired: 2 out]
        n178 = call-poly "Enqueue Message.vi"("Priority Message? (F)"=w435, "Message"=w436, "Message Queue"=w439) -> ()  [unwired: 7 in, 2 out]
        n179 = call-poly "Enqueue Message.vi"("Priority Message? (F)"=w435, "Message"=w436, "Message Queue"=w438) -> ()  [unwired: 7 in, 2 out]
        n180 = call-poly "Enqueue Message.vi"("Priority Message? (F)"=w435, "error in (no error)"=w424, "Message"=w436, "Message Queue"=w437) -> ("error out"=w433:errorcluster)  [unwired: 6 in, 1 out]
        n181 = Unbundle By Name(w419) -> ("Control references"=w428)
        n182 = Build Array("seguir" ("String")) -> (w425:string[])
        n183 = call-poly "get control reference by name.vi"("error in (no error)"=w433, "Control name"="guardar_Vref" ("String"), "Control references"=w428) -> ("error out"=w423:errorcluster, "Ctl Refnum"=w431:refnum<vi>)  [unwired: 3 in]
        n184 = Build Array(w431) -> (w430:refnum<vi>[])
        n185 = call-poly "get control reference by name.vi"("error in (no error)"=w423, "Control names"=w425, "Control references"=w428) -> ("error out"=w418:errorcluster, "References"=w427:refnum<vi>[])  [unwired: 3 in]
        n186 = call "Enable_Visible Buttons.vi"("Enable? (T)"=FALSE, "Controls Ref Array"=w430) -> ()  [unwired: 10 in]
        n187 = call "Enable_Visible Buttons.vi"("Enable? (T)"=TRUE, "Controls Ref Array"=w427) -> ()  [unwired: 10 in]
        n188 = local write "frecMon1"(w440) -> ()
        n189 = local write "voltMon1"(w440) -> ()
        n190 = local write "frecMon2"(w440) -> ()
        n191 = local write "voltMon2"(w440) -> ()
      }
      frame "guardaVref" {
        n192 = local read "AjusteAmp"() -> (w443:T1)
        "Vref" <- w443
        n193 = Number To Fractional String(number=w443, precision (6)=i16 3) -> (F-format string=w444:string)  [unwired: 2 in]
        n194 = Format Into String(format string="Se guardó Vref = %s volts", w444) -> (resulting string=w447:string)  [unwired: 2 in, 1 out]
        n195 = One Button Dialog(message=w447) -> ()  [unwired: 1 in, 1 out]
      }
      frame "guardaVref2" {
        n196 = local read "AjusteAmp2"() -> (w450:T1)
        "Vref2" <- w450
        n197 = Number To Fractional String(number=w450, precision (6)=i16 3) -> (F-format string=w451:string)  [unwired: 2 in]
        n198 = Format Into String(format string="Se guardó Vref = %s volts", w451) -> (resulting string=w454:string)  [unwired: 2 in, 1 out]
        n199 = One Button Dialog(message=w454) -> ()  [unwired: 1 in, 1 out]
      }
      frame "Error" {
        w462 = T10 1 items=["no dialog", "OK message", "continue or stop message", "OK message + warnings", "continue/stop + warnings"] ("type of dialog (OK msg:1)")
        n200 = Variant To Data(error in=w458, type=errorcluster {"status"=FALSE, "code"=0, "source"=""} ("error out"), Variant=w455) -> (data=w460:errorcluster, error out=w459:errorcluster)
        n201 = call <vilib>:"Simple Error Handler.vi"("type of dialog (OK msg:1)"=w462, "error in (no error)"=w460) -> ()  [unwired: 3 in, 5 out]
        n202 = call-poly "Enqueue Message.vi"("error in (no error)"=w459, "Message"="Exit", "Message Queue"=w457) -> ("error out"=w456:errorcluster)  [unwired: 7 in, 1 out]
      }
      frame "----------------------Controles----------------------" {
      }
      frame "Exit" {
        w467 = TRUE
        # "#evangelio Manda a cerrar el EHL"
        # "#evangelio Manda a cerrar todos los Loops"
        n203 = Release Queue(queue=w473, error in (no error)=w474) -> (error out=w478:errorcluster)  [unwired: 1 in, 2 out]
        n204 = Unbundle By Name(w469) -> ("Control references"=w479)
        n205 = for {
          tunnel: w472 -> [w482] mode=indexing
          tunnel: w470 -> [w481]
          tunnel: TRUE -> [w480]
          n206 = call-poly "Enqueue Message.vi"("Priority Message? (F)"=w480, "Message"=w481, "Message Queue"=w482) -> ()  [unwired: 7 in, 2 out]
        }
        n207 = call "Close All Ref.vi"("error in (no error)"=w478, "Control references"=w479) -> ("error out"=w476:errorcluster)  [unwired: 9 in]
        n208 = call "Fire User Event - Stop.vi"("error in (no error)"=w476, "Event Data"=w467, "User Event"="Exit EHL", "User Event in"=w471) -> ("error out"=w468:errorcluster)  [unwired: 7 in]
      }
      frame "Confirmar Salida" {
        n209 = Two Button Dialog(message="¿Quieres cerrar la aplicación?", 1:"No" ("T button name (\"OK\")"), 2:"Si" ("T button name (\"OK\")")) -> (T button?=w486:bool)
        n210 = case shown="True" w486 {
          tunnel: w485 -> [w491 w495]
          tunnel: [w491 w494] -> w483
          tunnel: w484 -> [_ w492]
          frame False {
          }
          frame True {
            n211 = call-poly "Enqueue Message.vi"("error in (no error)"=w495, "Message"="Exit", "Message Queue"=w492) -> ("error out"=w494:errorcluster)  [unwired: 7 in, 1 out]
          }
        }
      }
      frame Default {
        n212 = xnode "Error Ring"("parameter 0"=w497) -> ("error out"=w496:errorcluster)
      }
    }
    n213 = Unbundle By Name(w114) -> ("Tabla"=w113)
    n214 = call "Error Handler - Message Handling Loop.vi"("error in (no error)"=w104, "Message Queue"=w102) -> ("dup error in"=w103:errorcluster)  [unwired: 8 in, 1 out]
    n215 = local write "Tabla"(w113) -> ()
  }
  "Prueba09 out" <- w16
  n216 = call "Inst_CNT90.vi"("error in"=w1, "All Message Queues in"=w2, "Prueba31 in"=w3) -> ()  [unwired: 8 in, 1 out]
  n217 = call "Inst_DS360.vi"("error in"=w1, "All Message Queues in"=w2, "Prueba09 in"=w3) -> ()  [unwired: 8 in, 1 out]
  n218 = call "Inst_K2002.vi"("error in"=w1, "All Message Queues in"=w2, "Prueba31 in"=w3) -> ()  [unwired: 8 in, 1 out]
  n219 = Merge Errors(w18, w10) -> (→"error out":errorcluster)
